vi "Connect List.vi"(8 "error in (no error)":errorcluster, 10 "Params":variant, 11 "PIPXI40 Matrix in":refnum<class "PIPXI40 Matrix.lvclass">) -> (0 "error out":errorcluster, 3 "PIPXI40 Matrix out":refnum<class "PIPXI40 Matrix.lvclass">)   [LabVIEW 2020, in "PIPXI40.lvlib" / "PIPXI40 Matrix.lvclass"]
uses:
  PIPXI40 Matrix.lvclass
  D:/WSGitHub/RTFWK/Realization/PIPXI40 Base/PIPXI40 Base.lvclass
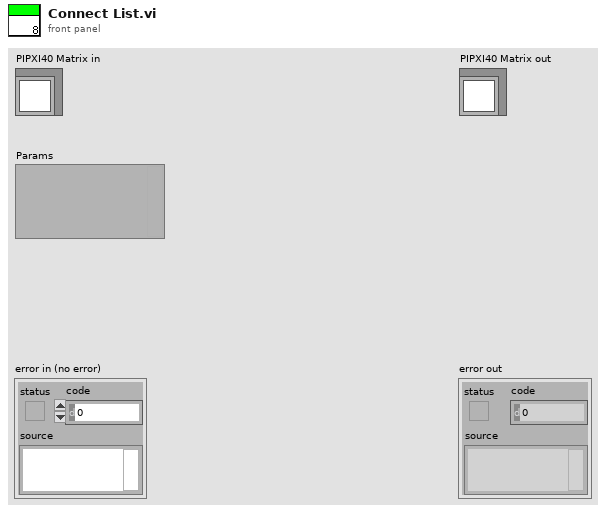
[diagram p1: front panel]
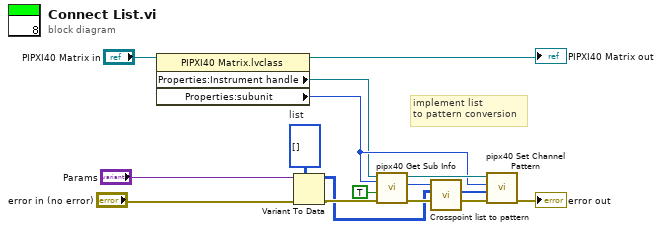
[diagram p0: block diagram]
diagram:
  w15 = i32[][] []  # list
  # "implement list\nto pattern conversion"
  n1 = property class="PIPXI40 Matrix.lvclass"(reference="PIPXI40 Matrix in") -> (reference out=→"PIPXI40 Matrix out":refnum<class "PIPXI40 Matrix.lvclass">, "Properties:Instrument handle"=w6:refnum<visa-resource-name>, "Properties:subunit"=w7:u32)  [unwired: 1 in, 1 out]
  n2 = Variant To Data(error in="error in (no error)", type=w15, Variant="Params") -> (data=w2:i32[][], error out=w8:errorcluster)
  n3 = call <instrlib>:"pipx40 Get Sub Info.vi"("error in (no error)"=w8, "is output"=TRUE, "subunit number"=w7, "instrument handle"=w6) -> ("error out"=w9:errorcluster, "rows"=w1:u32, "instrument handle out"=w10:refnum<visa-resource-name>)  [unwired: 3 in, 2 out]
  n4 = call "Crosspoint list to pattern.vi"("List"=w2, "rows"=w1) -> ("Pattern"=w3:u32[])  [unwired: 9 in]
  n5 = call <instrlib>:"pipx40 Set Channel Pattern.vi"("error in (no error)"=w9, "pattern"=w3, "subunit number"=w7, "instrument handle"=w10) -> ("error out"=→"error out":errorcluster)  [unwired: 6 in, 1 out]
